vi "String to U32 Array.vi"(1 "string":string="Hello work") -> (0 "Array":u32[](array[numeric]) format="%x")   [LabVIEW 2009]
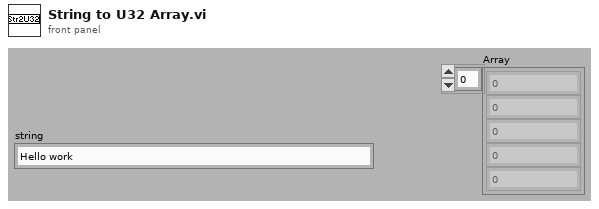
[diagram p1: front panel]
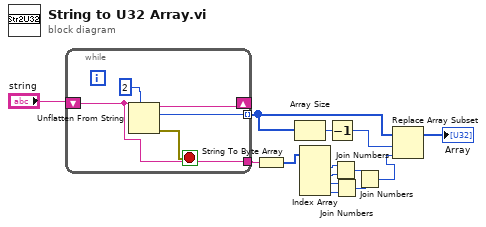
[diagram p0: block diagram]
diagram:
  n1 = while {
    shift-right: [w16] -> _
    shift-left: "string" -> [w15]
    tunnel: [w17] -> w4 mode=indexing
    tunnel: [w15] -> w6
    stop <- w18 stop-if-true
    n2 = Unflatten From String(type=u32 2 ("y"), binary string=w15) -> (rest of the binary string=w16:string, value=w17:u32, error out=w18:errorcluster)  [unwired: 1 in, 2 out]
  }
  n3 = String To Byte Array(string=w6) -> (unsigned byte array=w13:u8[])
  n4 = Array Size(array=w4) -> (size(s)=w5:i32)
  n5 = Index Array(array=w13) -> (element #1=w12:u8, element #2=w11:u8, element #3=w10:u8, element #4=w9:u8)  [unwired: 4 in]
  n6 = Decrement(x=w5) -> (x-1=w3:i32)
  n7 = Join Numbers(hi=w12, lo=w11) -> ((hi.lo)=w7:u16)
  n8 = Join Numbers(hi=w10, lo=w9) -> ((hi.lo)=w8:u16)
  n9 = Join Numbers(hi=w7, lo=w8) -> ((hi.lo)=w1:u32)
  n10 = Replace Array Subset(array=w4, new element=w1, index=w3) -> (→"Array":u32[])
